vi "g_AI InputsALB.vi"(7 "Action":enum16{"initialize", "read", "write"}(ring), 9 "AI in":dbl, 11 "Parameter":T2) -> (2 "AI out":T1)   [LabVIEW 2017]
uses:
  CtrlRefs/AnalogALB.ctl
  CtrlRefs/AnalogDisplayALB.ctl
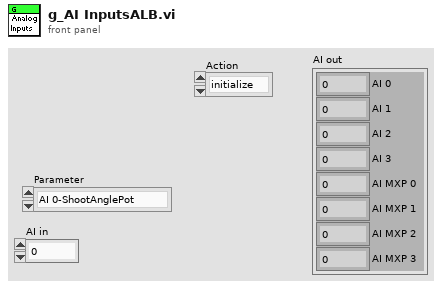
[diagram p1: front panel]
types:
  T1 = typedef "AnalogDisplayALB.ctl" = cluster{"AI 0":dbl, "AI 1":dbl, "AI 2":dbl, "AI 3":dbl, "AI MXP 0":dbl, "AI MXP 1":dbl, "AI MXP 2":dbl, "AI MXP 3":dbl}
  T2 = typedef "AnalogALB.ctl" = enum16{"AI 0-ShootAnglePot", "AI 1-TwrWallFlipPot", "AI 2-Sensor1Bk", "AI 3-Sonar", "AI MXP 0", "AI MXP 1", "AI MXP 2", "AI MXP 3"}
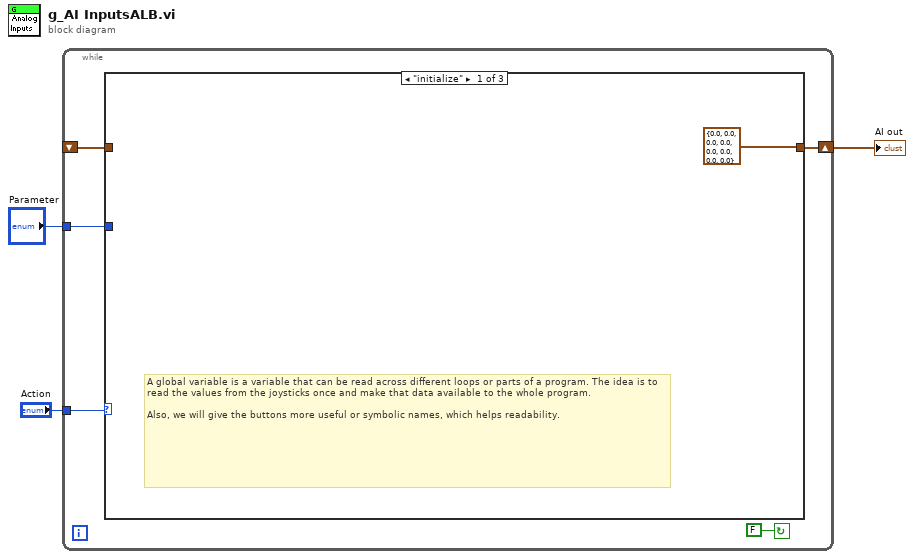
[diagram p0: block diagram]
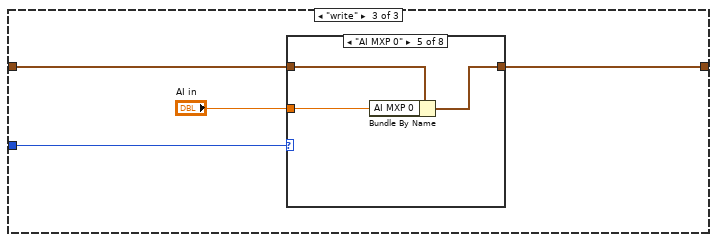
[diagram p3: hidden frame]
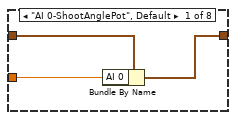
[diagram p4: hidden frame]
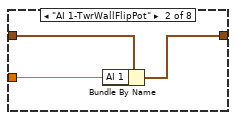
[diagram p5: hidden frame]
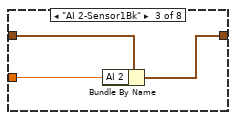
[diagram p6: hidden frame]
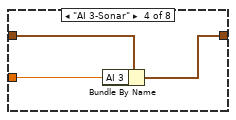
[diagram p7: hidden frame]
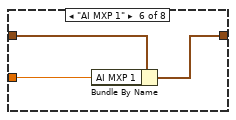
[diagram p8: hidden frame]
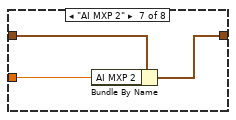
[diagram p9: hidden frame]
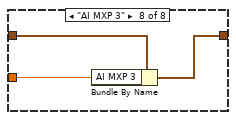
[diagram p10: hidden frame]
diagram:
  n1 = while {
    tunnel: "Action" -> [w7]
    shift-right: [w6] -> w1
    shift-left: _ -> [w5]
    tunnel: "Parameter" -> [w4]
    stop <- FALSE continue-if-true
    n2 = case shown="\"initialize\"" w7 {
      tunnel: [T1 {"AI 0"=0.0, "AI 1"=0.0, "AI 2"=0.0, "AI 3"=0.0, "AI MXP 0"=0.0, "AI MXP 1"=0.0, "AI MXP 2"=0.0, "AI MXP 3"=0.0} ("AI out") w10 w13] -> w6
      tunnel: w5 -> [_ w10 w14]
      tunnel: w4 -> [_ _ w12]
      frame "initialize" {
        # "A global variable is a variable that can be read across different loops or parts of a program. The idea is to read the values from the joysticks once and make that data available to the whole program.\n \nAlso, we will give the buttons more useful or symbolic names, which helps readability."
      }
      frame "read", Default {
      }
      frame "write" {
        n3 = case shown="\"AI MXP 0\"" w12 {
          tunnel: "AI in" -> [w15 w18 w21 w24 w27 w30 w33 w36]
          tunnel: w14 -> [w17 w20 w23 w26 w29 w32 w35 w38]
          tunnel: [w16 w19 w22 w25 w28 w31 w34 w37] -> w13
          frame "AI 0-ShootAnglePot", Default {
            n4 = Bundle By Name(cluster=w17, "AI 0"=w15) -> (w16:T1)
          }
          frame "AI 1-TwrWallFlipPot" {
            n5 = Bundle By Name(cluster=w20, "AI 1"=w18) -> (w19:T1)
          }
          frame "AI 2-Sensor1Bk" {
            n6 = Bundle By Name(cluster=w23, "AI 2"=w21) -> (w22:T1)
          }
          frame "AI 3-Sonar" {
            n7 = Bundle By Name(cluster=w26, "AI 3"=w24) -> (w25:T1)
          }
          frame "AI MXP 0" {
            n8 = Bundle By Name(cluster=w29, "AI MXP 0"=w27) -> (w28:T1)
          }
          frame "AI MXP 1" {
            n9 = Bundle By Name(cluster=w32, "AI MXP 1"=w30) -> (w31:T1)
          }
          frame "AI MXP 2" {
            n10 = Bundle By Name(cluster=w35, "AI MXP 2"=w33) -> (w34:T1)
          }
          frame "AI MXP 3" {
            n11 = Bundle By Name(cluster=w38, "AI MXP 3"=w36) -> (w37:T1)
          }
        }
      }
    }
  }
  "AI out" <- w1
